vi "Create and Register Sessions.vi"(8 "error in":errorcluster, 11 "sequence context":refnum<k7>) -> (0 "error out":errorcluster)   [LabVIEW 2020, in "NIDigitalSPI.lvlib"]
uses:
  NIDigitalSPI.lvlib
  <vilib>/MeasurementLink/MeasurementLink Session Management Client/RPC Messages/ni_measurementlink_PinMapContext.ctl
  <vilib>/MeasurementLink/MeasurementLink niDigital/Create Sessions - NSess.vi
  <vilib>/MeasurementLink/MeasurementLink Session Management Client/MeasurementLink Session Management Client.lvlib
  <vilib>/MeasurementLink/MeasurementLink TestStand Integration/MeasurementLink TestStand Integration.lvlib
  <vilib>/MeasurementLink/MeasurementLink Session Management/Session Reservation/Session Reservation.lvclass
  <vilib>/MeasurementLink/MeasurementLink niDigital/MeasurementLink niDigital.lvlib
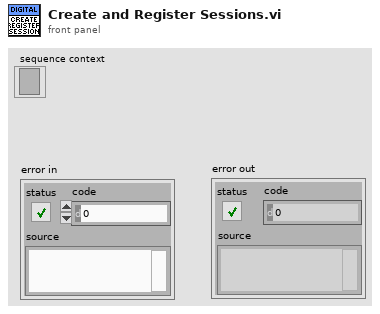
[diagram p1: front panel]
types:
  T1 = typedef "MeasurementLink Session Management Client.lvlib/ni_measurementlink_PinMapContext.ctl" = cluster{"pin_map_id":string, "sites":i32[]}
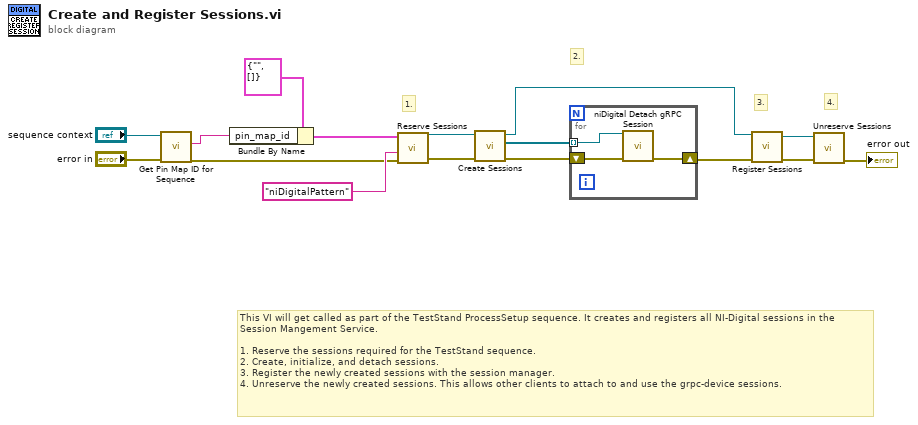
[diagram p0: block diagram]
diagram:
  # "1."
  # "2."
  # "3."
  # "4."
  # "This VI will get called as part of the TestStand ProcessSetup sequence. It creates and registers all NI-Digital sessions in the\nSession Mangement Service.\n\n1. Reserve the sessions required for the TestStand sequence. \n2. Create, initialize, and detach sessions.\n3. Register the newly created sessions with the session manager.\n4. Unreserve the newly created sessions. This allows other clients to attach to and use the grpc-device sessions."
  n1 = call <vilib>:"Get Pin Map ID for Sequence.vi"("error in"="error in", "sequence context in"="sequence context") -> ("error out"=w7:errorcluster, "pin map id"=w16:string)  [unwired: 7 in, 1 out]
  n2 = Bundle By Name(cluster=T1 {"pin_map_id"="", "sites"=[]} ("pin_map_context"), "pin_map_id"=w16) -> (w11:T1)
  n3 = call <vilib>:"Reserve Sessions.vi"("error in"=w7, "instrument type id"="niDigitalPattern" ("instrument_type_id"), "pin map context"=w11) -> ("error out"=w9:errorcluster, "session reservation out"=w10:refnum<class "Session Reservation.lvclass">)  [unwired: 7 in]
  n4 = call-poly <vilib>:"Create Sessions.vi"("error in"=w9, "session reservation in"=w10) -> ("error out"=w6:errorcluster, "sessions"=w5:refnum<k15>[], "session reservation out"=w4:refnum<class "Session Reservation.lvclass">)  [unwired: 6 in, 1 out]
  n5 = for {
    tunnel: w5 -> [w18] mode=indexing
    shift-right: [w17] -> w3
    shift-left: w6 -> [w19]
    n6 = call <instrlib>:"niDigital Detach gRPC Session.vi"("instrument handle"=w18, "error in"=w19) -> ("error out"=w17:errorcluster)  [unwired: 13 in]
  }
  n7 = call <vilib>:"Register Sessions.vi"("error in"=w3, "session reservation in"=w4) -> ("error out"=w2:errorcluster, "session reservation out"=w8:refnum<class "Session Reservation.lvclass">)  [unwired: 8 in]
  n8 = call <vilib>:"Unreserve Sessions.vi"("error in"=w2, "session reservation in"=w8) -> ("error out"=→"error out":errorcluster)  [unwired: 9 in]
